vi "GetPin.vi"(8 "error in (no error)":errorcluster, 9 "Pin":u8, 10 "Port":u8, 11 "NXP LPCXpresso54608 in":refnum<class "NXP LPCXpresso54608.lvclass">) -> (0 "error out":errorcluster, 1 "Response":string, 2 "Value":bool, 3 "NXP LPCXpresso54608 out":refnum<class "NXP LPCXpresso54608.lvclass">)   [LabVIEW 2020, in "NXP LPCXpresso54608.lvclass"]
doc: "Sends a command to read the pin status from the target device."
uses:
  NXP LPCXpresso54608.lvclass
  MCU/MCU.lvclass
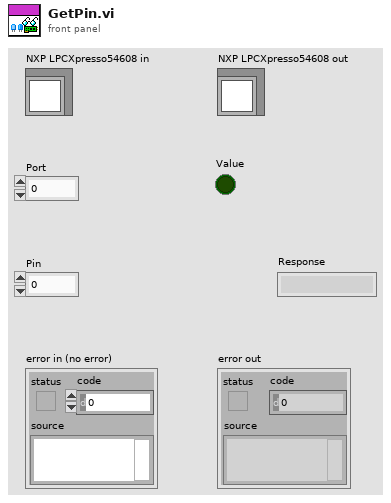
[diagram p1: front panel]
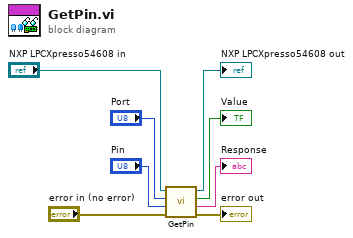
[diagram p0: block diagram]
diagram:
  n1 = call-parent "GetPin.vi"("error in (no error)"="error in (no error)", "Pin"="Pin", "Port"="Port", "MCU in"="NXP LPCXpresso54608 in") -> ("error out"=→"error out":errorcluster, "Response"=→"Response":string, "Value"=→"Value":bool, "MCU out"=→"NXP LPCXpresso54608 out":refnum<class "NXP LPCXpresso54608.lvclass">)  [unwired: 4 in]
